vi "Stimulus-Set Level (full wrapper).vi"(0 "Stimulus Channel":T25(xcontrol), 1 "Apply multiplier? (F)":bool, 5 "Waveform in":dbl[](array[numeric]), 11 "error in (no error)":errorcluster) -> (4 "Stimulus Channel out":T25(xcontrol), 6 "Waveform out":dbl[](array[numeric]), 8 "Multiplier":dbl, 10 "Ceiling":dbl, 15 "error out":errorcluster)   [LabVIEW 2020]
uses:
  Controls/Stimulus Channel (Full)/Stimulus Channel (Full).xctl
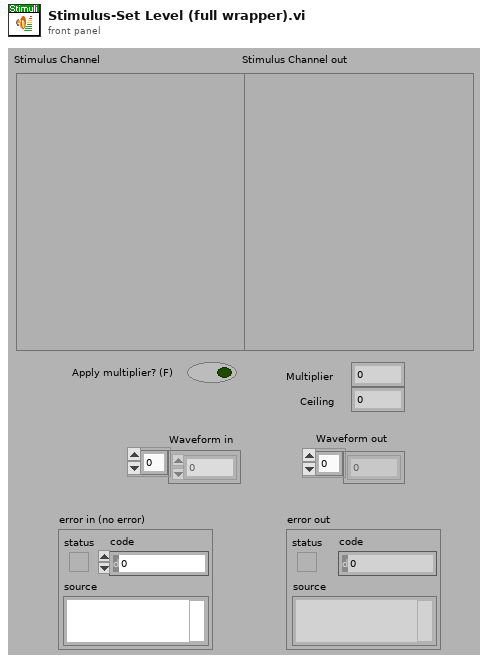
[diagram p1: front panel]
types:
  T1 = typedef "Waveform XCtl.xctl/Waveform Data.ctl" = cluster{"Type":T2, "Tone":T3, "Pulse Train":T4, "Noise":T7, "File":T8, "FMSweep":T9, "Chirp Train":T10, "Complex Tone":cluster{"Params":T12, "Data":T14}, "Moving Ripple":T15}
  T2 = typedef "Waveform Enum.ctl" = enum16{"OFF", "Tone", "Noise", "Pulse Train", "File", "FM Sweep", "Chirp Train", "Complex Tone", "FM Tone", "Moving Ripple"}
  T3 = typedef "Tone Params.ctl" = cluster{"Frequency (kHz)":dbl, "Last Freq":dbl, "Last Phase":dbl}
  T4 = typedef "Pulse Train Params.ctl" = cluster{"Pulse width (us)":dbl, "Pulse rate (Hz)":dbl, "Gap (ms)":dbl, "Polarity":T5, "PT State":T6, "Asynch":bool}
  T5 = typedef "Pulse Polarity.ctl" = enum16{"POS", "NEG", "POS-NEG", "NEG-POS"}
  T6 = typedef "PT-Continuous State.ctl" = cluster{"Template":dbl[], "Nperiod":i32, "Index":i32, "Pulse Rate (Hz)":dbl, "Phase (cycles)":dbl, "Noff":i32}
  T7 = typedef "Noise Params.ctl" = cluster{"InvFilt":bool, "Noise":dbl[], "CurPt":i32, "Aweight":bool, "Seed":i32, "afile":path}
  T8 = typedef "StimFile-Params.ctl" = cluster{"Filename":path, "Signal":dbl[], "Channel":i32, "stream":bool, "offset":i32, "nreps":i32, "loops":i32, "Randomize":bool, "order":i32[], "Seed":i32, "Tokens":i32}
  T9 = typedef "FM Sweep Params.ctl" = cluster{"Rate (oct/s)":dbl, "Fmin (Hz)":dbl, "Fmax (Hz)":dbl, "Ramp (ms)":dbl, "Linear":bool}
  T10 = typedef "Chirp Train.ctl" = cluster{"Params":T11, "Data":cluster{"WF":dbl[]}}
  T11 = typedef "Chirp Train Params.ctl" = cluster{"Fmin (kHz)":dbl, "Fmax (kHz)":dbl, "Compensate":bool, "Duration (ms)":dbl}
  T12 = typedef "CT-Params.ctl" = cluster{"F0 (Hz)":dbl, "Band":cluster{"Flow (Hz)":dbl, "Fhigh (Hz)":dbl}, "Phase":T13, "Min F0 (Hz)":dbl, "Max F0 (Hz)":dbl, "ContinRandPhase":bool, "Max peak factor":dbl, "Max mod depth":dbl, "MinHarmNum":i32, "MaxHarmNum":i32, "Level Mode":enum16{"per component", "overall rms"}, "% jitter":dbl}
  T13 = typedef "CT-Phase Enum.ctl" = enum16{"Cosine", "Random", "Alternating"}
  T14 = typedef "CT-Runtime Data.ctl" = cluster{"Ncomp":i32, "MinHarm":i32, "Phase":dbl[], "Amplitude":dbl[], "Npts/frame":i32, "Last F0":dbl, "Fmin":dbl, "Fmax":dbl, "Lslope":dbl, "randphase":bool, "overall rms":bool, "fmult":dbl[], "jittered":bool}
  T15 = typedef "Moving Ripple.ctl" = cluster{"Params":T16, "Data":T17}
  T16 = typedef "Moving Ripple.Params.ctl" = cluster{"Fmin":dbl, "Fmax":dbl, "Density":dbl, "Velocity":dbl, "Depth":dbl, "Phase":dbl, "Comp/oct":i32}
  T17 = typedef "Moving Ripple.Data.ctl" = cluster{"Freq":dbl[], "A":dbl[], "phase":dbl[], "Phase":dbl}
  T18 = typedef "Advanced Filter XCtl.xctl/Filter Data.ctl" = cluster{"Type":enum16{"Lowpass", "Highpass", "Bandpass", "Bandstop", "OFF"}, "CF (kHz)":dbl, "BW (kHz)":dbl, "Cascade":bool, "Quadrature":bool, "Scale Factor":dbl, "Stages":cluster{"IIR Filter":cluster{"filter structure":enum32{"IIR 2nd Order", "IIR 4th Order"}, "Reverse Coefficients":dbl[], "Forward Coefficients":dbl[]}, "State":dbl[]}[], "Class":enum16{"Elliptic", "Butterworth"}, "Order":i32, "BWUnits":T19}
  T19 = typedef "Filter-Bandwidth Units.ctl" = enum16{"Linear", "Octaves", "Min-Max"}
  T20 = typedef "Burst Control.xctl/Burst Data.ctl" = cluster{"Active":bool, "Delay (ms)":dbl, "Duration (ms)":dbl, "Ramp (ms)":dbl, "Rate (Hz)":dbl, "Trepeat (ms)":dbl, "Repeat":bool}
  T21 = typedef "Level XCtl.xctl/Level Data.ctl" = cluster{"Level":dbl, "Units":T22, "Max":dbl, "Multiplier":dbl, "Cal File":path, "Cal":cluster{"Freq (Hz)":dbl[], "Mag (dB SPL)":dbl[], "Phase (deg)":dbl[]}}
  T22 = typedef "Level Units.ctl" = enum16{"dB atten", "dB SPL", "dB re 1 Vrms", "dB V/Hz½", "mW", "dB HL", "Volts", "dB mW"}
  T23 = typedef "Advanced Stimulus Options.xctl/Advanced Stimulus Options.ctl" = cluster{"Rep Mask":string, "AltPol":bool, "Var":string, "Expr":string, "Persist":bool}
  T24 = typedef "SAM Params.ctl" = cluster{"Active":bool, "Frequency (Hz)":dbl, "Depth":dbl, "Init Phase (cycles)":dbl, "phase (degrees)":dbl, "Asynch":bool}
  T25 = cluster{"Waveform":T1, "Filter":T18, "Burst":T20, "Level":T21, "Name":string, "Advanced":T23, "SAM":T24}
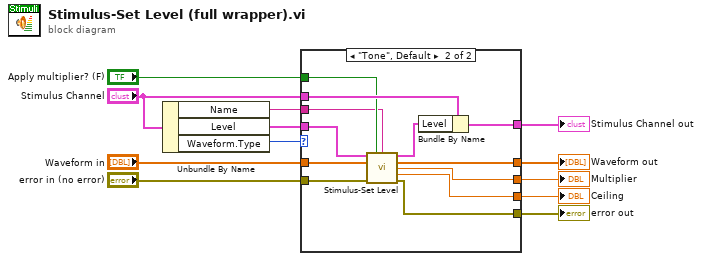
[diagram p0: block diagram]
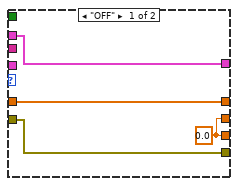
[diagram p2: hidden frame]
diagram:
  n1 = Unbundle By Name("Stimulus Channel") -> ("Name"=w2:string, "Level"=w10:T21, "Waveform.Type"=w1:T2)
  n2 = case shown="\"Tone\", Default" w1 {
    tunnel: "Waveform in" -> [w14 w28]
    tunnel: "error in (no error)" -> [w15 w27]
    tunnel: w10 -> [_ w26]
    tunnel: [w16 w25] -> w9
    tunnel: "Stimulus Channel" -> [w16 w24]
    tunnel: [w14 w22] -> w7
    tunnel: "Apply multiplier? (F)" -> [_ w21]
    tunnel: [w13 w20] -> w5
    tunnel: [w13 w19] -> w4
    tunnel: [w15 w18] -> w3
    tunnel: w2 -> [_ w17]
    frame "OFF" {
      w13 = 0.0 ("Ceiling")
    }
    frame "Tone", Default {
      n3 = call "Stimulus-Set Level.vi"("Level"=w26, "Apply multiplier? (F)"=w21, "Name"=w17, "Waveform in"=w28, "error in (no error)"=w27) -> ("Level out"=w23:T21, "Waveform out"=w22:dbl[], "Multiplier"=w20:dbl, "Ceiling"=w19:dbl, "error out"=w18:errorcluster)  [unwired: 6 in]
      n4 = Bundle By Name(cluster=w24, "Level"=w23) -> (w25:T25)
    }
  }
  "error out" <- w3
  "Stimulus Channel out" <- w9
  "Waveform out" <- w7
  "Multiplier" <- w5
  "Ceiling" <- w4
